vi "CSM - Request CSM to Broadcast Status Change.vi"(4 "Immediately?(F)":bool, 6 "Broadcast(T)":bool=TRUE, 7 "Module Name":string, 8 "Error In (no error)":errorcluster, 10 "Arguments (\"\")":string, 11 "Status":string="DoA") -> (0 "error out":errorcluster)   [LabVIEW 2020, in "Communicable State Machine.lvlib"]
doc: "Request CSM to publish status change to CSM specified. This is usually used in sub-loops with a CSM for acting as a holistic module.\n\n<b>Inputs:</b>\n - <b>Status</b>: status to broadcast.\n - <b>Arguments (\"\")</b>: Argument of the status.\n - <b>Module Name</b>:Host Module Name\n - <b>Broadcast(T)</b>: Trigger for broadcast or not.\n - <b>Error In (no error)</b>: Error cluster\n\n<b>Outputs:</b>\n - <b>error out</b>: Error cluster"
uses:
  Communicable State Machine.lvlib
  _CSM_MSG_TYPE.ctl
  _Cross CSM State Data.ctl
  _Cross CSM State Response.ctl
  _CSM_Response Source Message.ctl
  _CSMOFGVOPER.ctl
  Priority Queue.lvclass/Priority Queue.ctl
  Priority Queue.lvclass
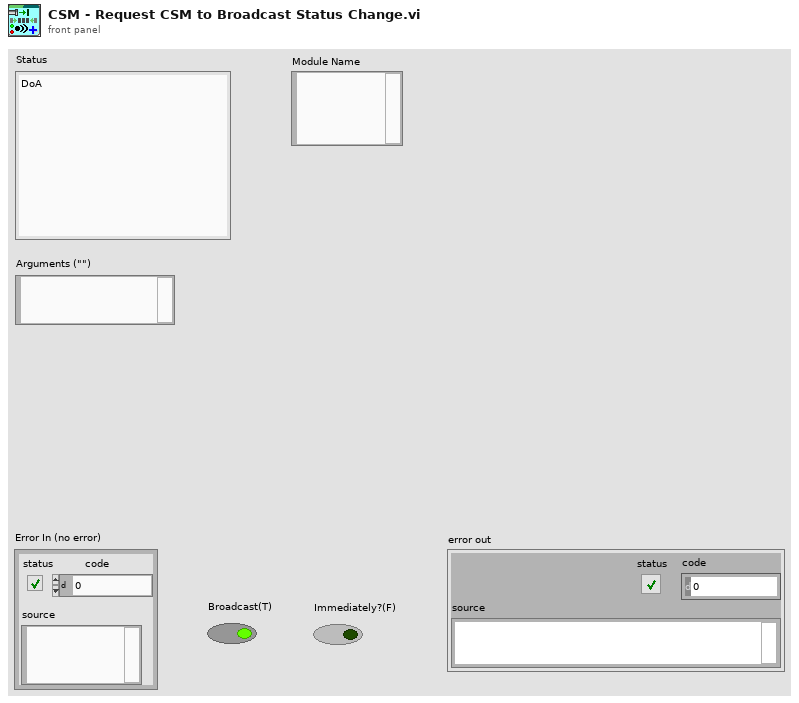
[diagram p1: front panel]
types:
  T1 = typedef "Communicable State Machine.lvlib/_CSM_MSG_TYPE.ctl" = enum16{"Sync Message(-@)", "Async Message(->)", "Async without Response(->|)", "Async Response", "Broadcast(-><all>)", "Broadcast(-><status>)", "Broadcast(-><interrupt>)", "Append to JKISM States", "Append to JKISM States(High Priority)"}
  T2 = typedef "Communicable State Machine.lvlib/_Cross CSM State Data.ctl" = cluster{"Msg Type":T1, "state":string, "args":string, "source":string, "RespQ":refnum<queue>, "Response For Message":T3, "Target":string}
  T3 = typedef "Communicable State Machine.lvlib/_CSM_Response Source Message.ctl" = cluster{"‘State":string, "’Arguments":string, "’Error":errorcluster}
  T4 = typedef "Communicable State Machine.lvlib/_CSMOFGVOPER.ctl" = enum16{"Create If not Exist", "Get By Name", "List", "Check If Name Exists", "Release", "Module Status", "Create Status Event Handler", "Destroy Status Event Handler"}
  T5 = typedef "Communicable State Machine.lvlib/_CSMObj.ctl" = cluster{"Requested Name":string, "Module Name":string, "Mode":T6, "Queue":refnum<class "Priority Queue.lvclass">, "CSM-Data":refnum<data-value>, "User Event":refnum<user-event>, "Status Change Event":refnum<user-event>, "Allowed Messages":string[], "Mode-Data":refnum<data-value>, "Group Name":string, "Exit Event":refnum<user-event>}
  T6 = typedef "Communicable State Machine.lvlib/_CSM_MODE.ctl" = enum16{"Not Exist", "Stand Alone", "CSM", "Worker Agent", "Worker", "Chain", "Chain Node"}
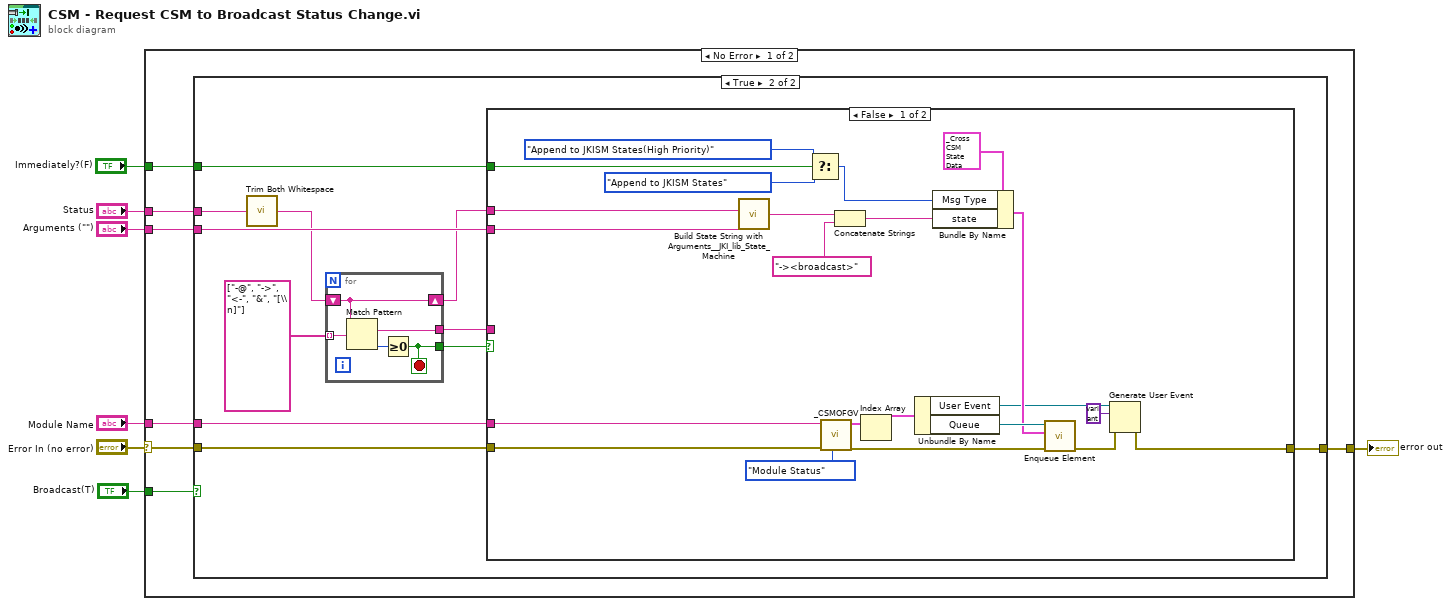
[diagram p0: block diagram]
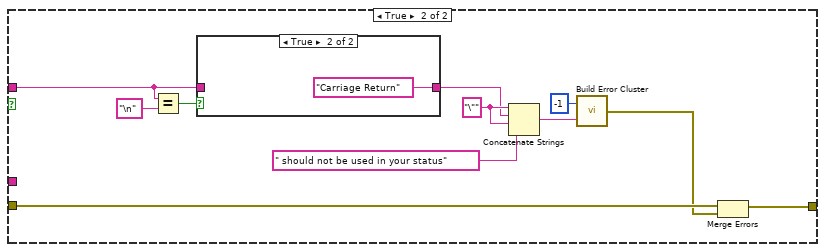
[diagram p3: hidden frame]
diagram:
  n1 = case shown="No Error" "Error In (no error)" {
    selector: "Error In (no error)" -> [w13 w67]
    tunnel: "Status" -> [w11 _]
    tunnel: [w14 w67] -> w5
    tunnel: "Arguments (\"\")" -> [w12 _]
    tunnel: "Module Name" -> [w10 _]
    tunnel: "Broadcast(T)" -> [w9 _]
    tunnel: "Immediately?(F)" -> [w8 _]
    frame No Error {
      n2 = case shown="True" w9 {
        tunnel: [w15 w26] -> w14
        tunnel: w13 -> [w15 w25]
        tunnel: w12 -> [_ w24]
        tunnel: w11 -> [_ w23]
        tunnel: w10 -> [_ w22]
        tunnel: w8 -> [_ w16]
        frame False {
        }
        frame True {
          n3 = call "Trim Both Whitespace.vi"("string"=w23) -> ("trimmed string"=w17:string)  [unwired: 1 in]
          n4 = for {
            shift-right: [w66] -> w20
            shift-left: w17 -> [w66]
            tunnel: string[] ["-@", "->", "<-", "&", "[\\n]"] -> [w65] mode=indexing
            tunnel: [w63] -> w18
            tunnel: [w62] -> w19
            stop <- w62 stop-if-true
            n5 = Match Pattern(string=w66, regular expression=w65) -> (match substring=w63:string, offset past match=w64:i32)  [unwired: 1 in, 2 out]
            n6 = Greater Or Equal To 0?(x=w64) -> (x >= 0?=w62:bool)
          }
          n7 = case shown="False" w19 {
            tunnel: w24 -> [w28 _]
            tunnel: [w36 w51] -> w26
            tunnel: w25 -> [w41 w52]
            tunnel: w20 -> [w29 _]
            tunnel: w18 -> [_ w49]
            tunnel: w22 -> [w40 _]
            tunnel: w16 -> [w35 _]
            frame False {
              n8 = call "Build State String with Arguments__JKI_lib_State_Machine.vi"("Arguments (\"\")"=w28, "State"=w29) -> ("State with Arguments"=w30:string)  [unwired: 4 in]
              n9 = Select(t=_CSM_MSG_TYPE."Append to JKISM States(High Priority)" ("Msg Type"), s=w35, f=_CSM_MSG_TYPE."Append to JKISM States" ("Msg Type")) -> (s? t:f=w32:T1)
              n10 = call "_CSMOFGV.vi"("Operation"=_CSMOFGVOPER."Module Status", "Error in"=w41, "Name(\"\" to use uuid) in"=w40) -> ("Error out"=w42:errorcluster, "Array"=w47:T5[])  [unwired: 6 in, 1 out]
              n11 = Concatenate Strings(w30, "-><broadcast>" ("string")) -> (w27:string)
              n12 = Index Array(array=w47) -> (element=w46:T5)  [unwired: 1 in]
              n13 = Unbundle By Name(w46) -> ("User Event"=w38:refnum<user-event>, "Queue"=w45:refnum<class "Priority Queue.lvclass">)
              n14 = Bundle By Name(cluster=T2 {"Msg Type"=enum."Sync Message(-@)", "state"="", "args"="", "source"="", "RespQ"=refnum, "Response For Message"={"‘State"="", "’Arguments"="", "’Error"={"status"=FALSE, "code"=0, "source"=""}}, "Target"=""} ("element"), "Msg Type"=w32, "state"=w27) -> (w43:T2)
              n15 = call "Enqueue Element.vi"("error in (no error)"=w42, "Cross JKI State Machine State"=w43, "Priority Queue"=w45) -> ("error out"=w37:errorcluster)  [unwired: 7 in, 1 out]
              n16 = Generate User Event(user event=w38, event data cluster=variant ("event data"), error in=w37) -> (error out=w36:errorcluster)  [unwired: 1 in, 1 out]
            }
            frame True {
              w56 = "\"" ("string")
              n17 = Equal?(x=w49, y="\n" ("regular expression")) -> (x = y?=w53:bool)
              n18 = case shown="True" w53 {
                tunnel: [w60 "Carriage Return" ("State")] -> w55
                tunnel: w49 -> [w60 _]
                frame False {
                }
                frame True {
                }
              }
              n19 = Concatenate Strings(w56, w55, w56, " should not be used in your status" ("String to Prepend to source (\"\")")) -> (w57:string)
              n20 = call "Build Error Cluster.vi"("String to Prepend to source (\"\")"=w57, "code"=-1) -> ("error out"=w50:errorcluster)
              n21 = Merge Errors(w52, w50) -> (w51:errorcluster)
            }
          }
        }
      }
    }
    frame Error {
    }
  }
  "error out" <- w5
